vi "基础价格.vi"(8 "error in (no error)":errorcluster caption="错误输入（无错误）", 11 "燕麦巧克力 输入":refnum<class "燕麦巧克力.lvclass">) -> (0 "error out":errorcluster caption="错误输出", 2 "基础价格":dbl, 3 "燕麦巧克力 输出":refnum<class "燕麦巧克力.lvclass">)   [LabVIEW 2016, in "燕麦巧克力.lvclass"]
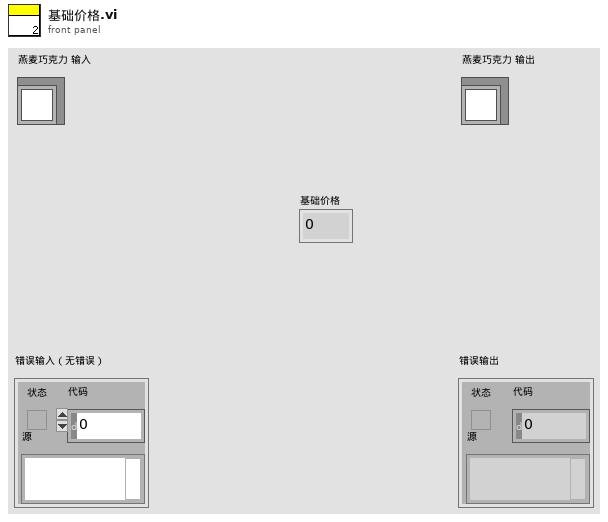
[diagram p1: front panel]
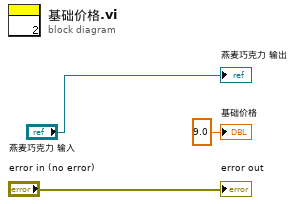
[diagram p0: block diagram]
diagram:
  "error out" <- "error in (no error)"
  "燕麦巧克力 输出" <- "燕麦巧克力 输入"
  "基础价格" <- 9.0 ("基础价格")
